vi "Error Query.vi"(8 "error in (no error)":errorcluster, 11 "VISA resource name":refnum<visa-resource-name>) -> (0 "error out":errorcluster, 1 "Error Message":string, 2 "Error":i32, 3 "VISA resource name out":refnum<visa-resource-name>)   [LabVIEW 2016, in "Agilent 428X Series.lvlib"]
doc: "This VI reads an error from the instrument. It expects to see errors in SCPI format (#,\"error message\")."
uses:
  <instrlib>/Agilent 428X Series/Agilent 428X Series.lvlib
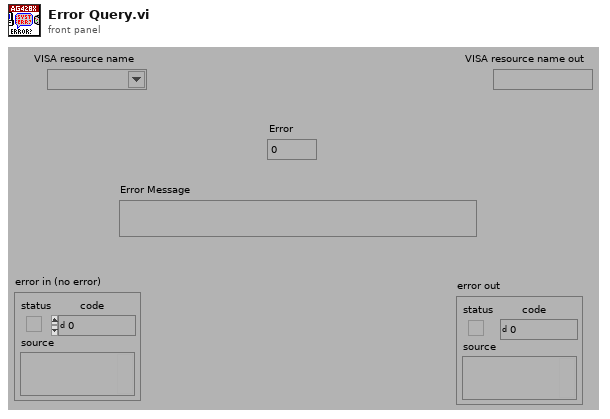
[diagram p1: front panel]
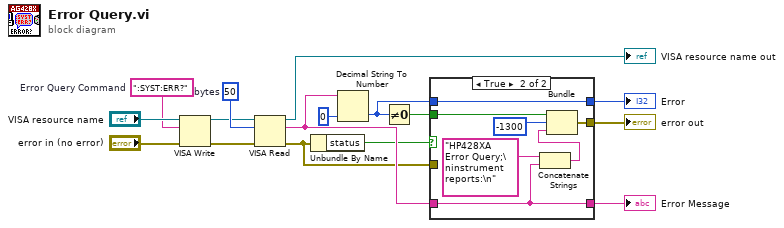
[diagram p0: block diagram]
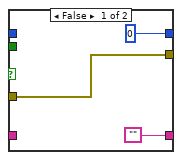
[diagram p2: hidden frame]
diagram:
  w5 = u32 50  # bytes
  w7 = ":SYST:ERR?"  # Error Query Command
  n1 = VISA Write(VISA resource name="VISA resource name", write buffer=w7, error in (no error)="error in (no error)") -> (VISA resource name out=w4:refnum<visa-resource-name>, error out=w6:errorcluster)  [unwired: 1 out]
  n2 = VISA Read(VISA resource name=w4, byte count=w5, error in (no error)=w6) -> (VISA resource name out=→"VISA resource name out":refnum<visa-resource-name>, read buffer=w10:string, error out=w3:errorcluster)  [unwired: 1 out]
  n3 = Unbundle By Name(w3) -> ("status"=w8:bool)
  n4 = Decimal String To Number(string=w10, default (0L)=0) -> (number=w2:i32)  [unwired: 1 in, 1 out]
  n5 = Not Equal To 0?(x=w2) -> (x != 0?=w9:bool)
  n6 = case shown="True" w8 {
    tunnel: w10 -> [_ w24]
    tunnel: w3 -> [w19 _]
    tunnel: [w19 w22] -> w11
    tunnel: ["" w24] -> w16
    tunnel: [0 w21] -> w15
    tunnel: w2 -> [_ w21]
    tunnel: w9 -> [_ w20]
    frame False {
    }
    frame True {
      n7 = Concatenate Strings("HP428XA Error Query;\ninstrument reports:\n", w24) -> (w23:string)
      n8 = Bundle(w20, -1300, w23) -> (w22:errorcluster)  [unwired: 1 in]
    }
  }
  "Error Message" <- w16
  "Error" <- w15
  "error out" <- w11
